vi "GetSubimg.vi"(1 "width":u16, 2 "Img in":u16[][](array[numeric]), 3 "y":u16, 4 "x":u16, 5 "y_start":u16, 6 "x_start":u16) -> (0 "SubImage":u16[][](array[numeric]))   [LabVIEW 2012]
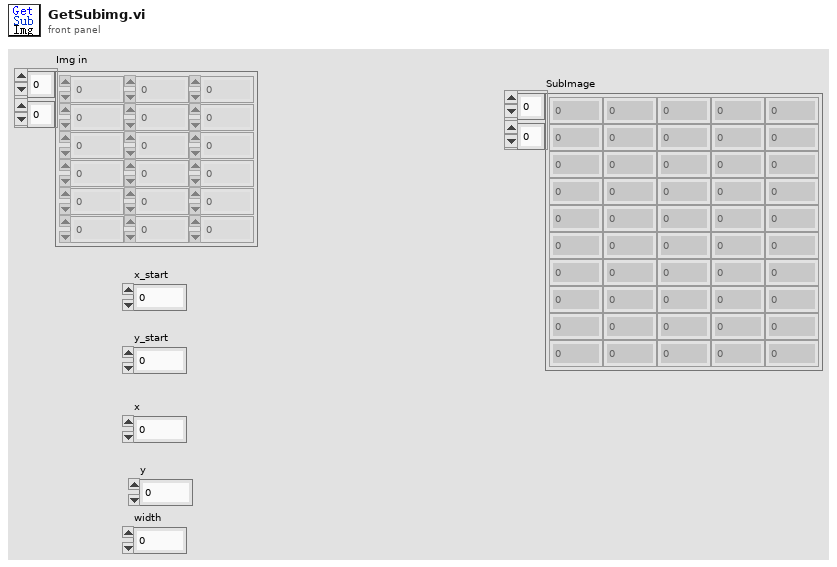
[diagram p1: front panel]
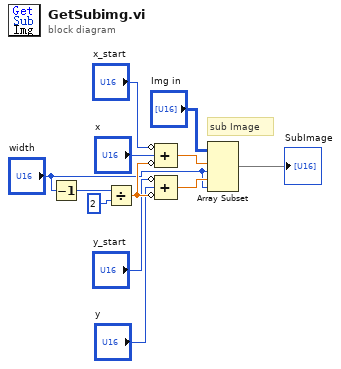
[diagram p0: block diagram]
diagram:
  # "sub Image"
  n1 = Decrement(x="width") -> (x-1=w10:u16)
  n2 = Divide(x=w10, y=u16 2) -> (x/y=w8:dbl)
  n3 = Compound Arithmetic op=ADD(invert "x_start", "x", invert w8) -> (w12:dbl)
  n4 = Compound Arithmetic op=ADD(invert "y_start", "y", invert w8) -> (w11:dbl)
  n5 = Array Subset(array="Img in", index (row)=w12, length (row)="width", index (col)=w11, length (col)="width") -> (→"SubImage":u16[][])
